vi "Read_uC_Data.vi"(8 "error in (no error)":errorcluster, 10 "String":string, 11 "VISA Refnum in":refnum<visa-resource-name>) -> (1 "VISA Refnum in 2":refnum<visa-resource-name>, 2 "Array":i32[](array[numeric]), 3 "SpecParamReceived":string)   [LabVIEW 2020]
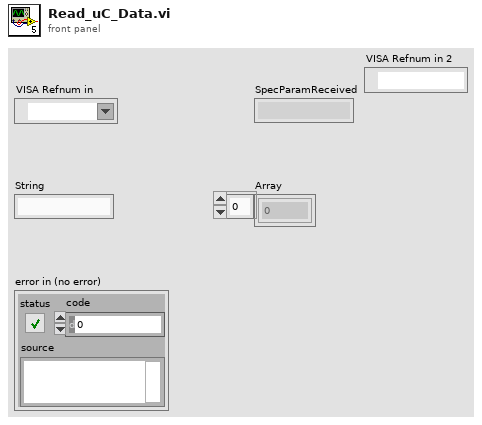
[diagram p1: front panel]
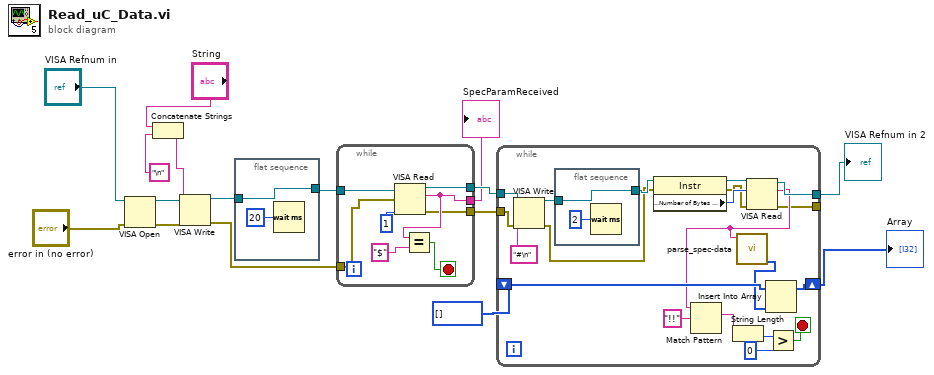
[diagram p0: block diagram]
diagram:
  n1 = VISA Open(error in (no error)="error in (no error)", VISA resource name="VISA Refnum in") -> (VISA resource name=w6:refnum<visa-resource-name>, error out=w5:errorcluster)  [unwired: 3 in]
  n2 = Concatenate Strings("String", "\n") -> (w10:string)
  n3 = VISA Write(VISA resource name=w6, write buffer=w10, error in (no error)=w5) -> (VISA resource name out=w7:refnum<visa-resource-name>, error out=w9:errorcluster)  [unwired: 1 out]
  n4 = flat-sequence {
    tunnel: [w18] -> w8
    tunnel: w7 -> [w18]
    frame #0 {
      n5 = Wait (ms)(milliseconds to wait=u32 20) -> ()  [unwired: 1 out]
    }
  }
  n6 = while {
    tunnel: w8 -> [w24]
    tunnel: w9 -> [w25]
    tunnel: [w22] -> w13
    tunnel: [w20] -> w14
    tunnel: [w19] -> w2
    stop <- w21 stop-if-true
    n7 = VISA Read(VISA resource name=w24, byte count=u32 1, error in (no error)=w25) -> (VISA resource name out=w20:refnum<visa-resource-name>, read buffer=w22:string, error out=w19:errorcluster)  [unwired: 1 out]
    n8 = Equal?(x=w22, y="$") -> (x = y?=w21:bool)
  }
  "SpecParamReceived" <- w13
  n9 = while {
    tunnel: w14 -> [w46]
    tunnel: [w40] -> w1
    shift-right: [w37] -> w16
    shift-left: i32[] [] -> [w39]
    tunnel: w2 -> [w30]
    tunnel: [w27] -> _
    stop <- w31 stop-if-true
    n10 = VISA Write(VISA resource name=w46, write buffer="#\n", error in (no error)=w30) -> (VISA resource name out=w44:refnum<visa-resource-name>, error out=w29:errorcluster)  [unwired: 1 out]
    n11 = flat-sequence {
      tunnel: [w48] -> w41
      tunnel: w44 -> [w48]
      frame #0 {
        n12 = Wait (ms)(milliseconds to wait=u32 2) -> ()  [unwired: 1 out]
      }
    }
    n13 = property class="Instr"(reference=w41, error in=w29) -> (reference out=w43:refnum<visa-resource-name>, error out=w28:errorcluster, "Serial Settings:Number of Bytes at Serial Port"=w42:u32)
    n14 = VISA Read(VISA resource name=w43, byte count=w42, error in (no error)=w28) -> (VISA resource name out=w40:refnum<visa-resource-name>, read buffer=w36:string, error out=w27:errorcluster)  [unwired: 1 out]
    n15 = Match Pattern(string=w36, regular expression="!!") -> (match substring=w34:string)  [unwired: 1 in, 3 out]
    n16 = String Length(string=w34) -> (length=w33:i32)
    n17 = call "parse_spec-data.vi"("String"=w36) -> ("Array 2"=w38:u16[])  [unwired: 10 in]
    n18 = Insert Into Array(array=w39, new element=w38) -> (w37:i32[])  [unwired: 1 in]
    n19 = Greater?(x=w33, y=0) -> (0:w31:bool)
  }
  "Array" <- w16
  "VISA Refnum in 2" <- w1
